vi "StringParser.vi"(0 "Input":string) -> (1 "R/W":string, 2 "Port (Port 1)":T2 items=["Port 1", "Port 2", "Port 3", "Port 4"], 3 "Output Port (All Ports)":T1=3 items=["Port A"=0, "Port B"=1, "Port C"=2, "Ports A & B"=4, "Ports A & C"=5, "Ports B & C"=6, "All Ports"=3], 4 "NewValue":i32)   [LabVIEW 2013]
uses:
  <vilib>/NXT/Block Support/NXT_InputPort.ctl
  <vilib>/NXT/Subs/MotorOutput.ctl
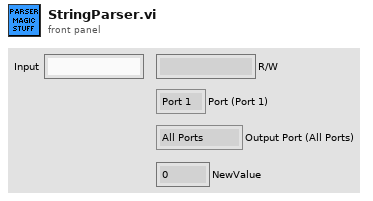
[diagram p1: front panel]
types:
  T1 = typedef "MotorOutput.ctl" = u8
  T2 = typedef "NXT_InputPort.ctl" = u32
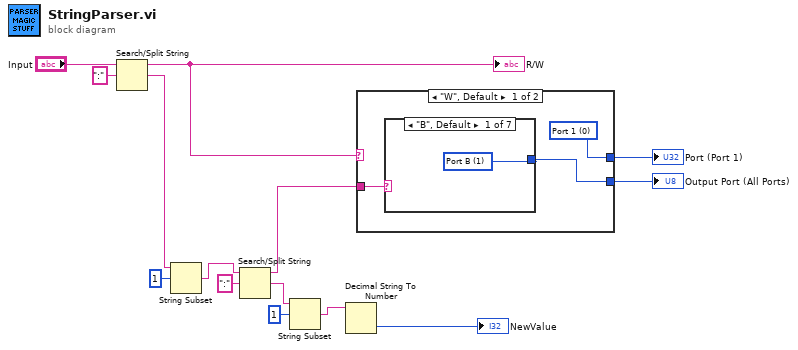
[diagram p0: block diagram]
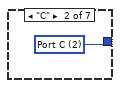
[diagram p2: hidden frame]
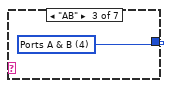
[diagram p3: hidden frame]
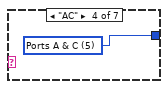
[diagram p4: hidden frame]
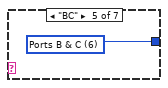
[diagram p5: hidden frame]
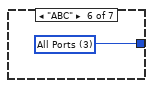
[diagram p6: hidden frame]
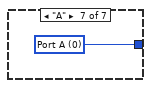
[diagram p7: hidden frame]
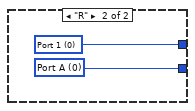
[diagram p8: hidden frame]
diagram:
  n1 = Search/Split String(string="Input", search string/char (-)=":") -> (substring before match=w5:string, match + rest of string=w4:string)  [unwired: 1 in, 1 out]
  "R/W" <- w5
  n2 = String Subset(string=w4, offset (0)=1) -> (substring=w9:string)  [unwired: 1 in]
  n3 = Search/Split String(string=w9, search string/char (-)=":") -> (substring before match=w1:string, match + rest of string=w7:string)  [unwired: 1 in, 1 out]
  n4 = String Subset(string=w7, offset (0)=1) -> (substring=w6:string)  [unwired: 1 in]
  n5 = Decimal String To Number(string=w6) -> (number=→"NewValue":i32)  [unwired: 2 in, 1 out]
  n6 = case shown="\"W\", Default" w5 {
    tunnel: [w17 w26] -> w3
    tunnel: [w16 w25] -> w2
    tunnel: w1 -> [w15 _]
    frame "W", Default {
      w16 = T2 0 items=["Port 1", "Port 2", "Port 3", "Port 4"] ("Port (Port 1)")
      n7 = case shown="\"B\", Default" w15 {
        tunnel: [w18 w19 w20 w21 w22 w23 w24] -> w17
        frame "B", Default {
          w18 = T1 1 items=["Port A"=0, "Port B"=1, "Port C"=2, "Ports A & B"=4, "Ports A & C"=5, "Ports B & C"=6, "All Ports"=3] ("Output Port (All Ports)")
        }
        frame "C" {
          w19 = T1 2 items=["Port A"=0, "Port B"=1, "Port C"=2, "Ports A & B"=4, "Ports A & C"=5, "Ports B & C"=6, "All Ports"=3] ("Output Port (All Ports)")
        }
        frame "AB" {
          w20 = T1 4 items=["Port A"=0, "Port B"=1, "Port C"=2, "Ports A & B"=4, "Ports A & C"=5, "Ports B & C"=6, "All Ports"=3] ("Output Port (All Ports)")
        }
        frame "AC" {
          w21 = T1 5 items=["Port A"=0, "Port B"=1, "Port C"=2, "Ports A & B"=4, "Ports A & C"=5, "Ports B & C"=6, "All Ports"=3] ("Output Port (All Ports)")
        }
        frame "BC" {
          w22 = T1 6 items=["Port A"=0, "Port B"=1, "Port C"=2, "Ports A & B"=4, "Ports A & C"=5, "Ports B & C"=6, "All Ports"=3] ("Output Port (All Ports)")
        }
        frame "ABC" {
          w23 = T1 3 items=["Port A"=0, "Port B"=1, "Port C"=2, "Ports A & B"=4, "Ports A & C"=5, "Ports B & C"=6, "All Ports"=3] ("Output Port (All Ports)")
        }
        frame "A" {
          w24 = T1 0 items=["Port A"=0, "Port B"=1, "Port C"=2, "Ports A & B"=4, "Ports A & C"=5, "Ports B & C"=6, "All Ports"=3] ("Output Port (All Ports)")
        }
      }
    }
    frame "R" {
      w25 = T2 0 items=["Port 1", "Port 2", "Port 3", "Port 4"] ("Port (Port 1)")
      w26 = T1 0 items=["Port A"=0, "Port B"=1, "Port C"=2, "Ports A & B"=4, "Ports A & C"=5, "Ports B & C"=6, "All Ports"=3] ("Output Port (All Ports)")
    }
  }
  "Port (Port 1)" <- w2
  "Output Port (All Ports)" <- w3
